vi "SACB - 1.vi"(6 "RH?":bool, 7 "Command":enum16{"Create", "Read", "Close"}(ring), 8 "Error In":errorcluster) -> (0 "Error Out":errorcluster, 3 "Digital Inputs":T1)   [LabVIEW 2017]
uses:
  <vilib>/Modbus/master/Modbus Master.lvclass
  <vilib>/Modbus/master/Create Master Instance (TCP).vi
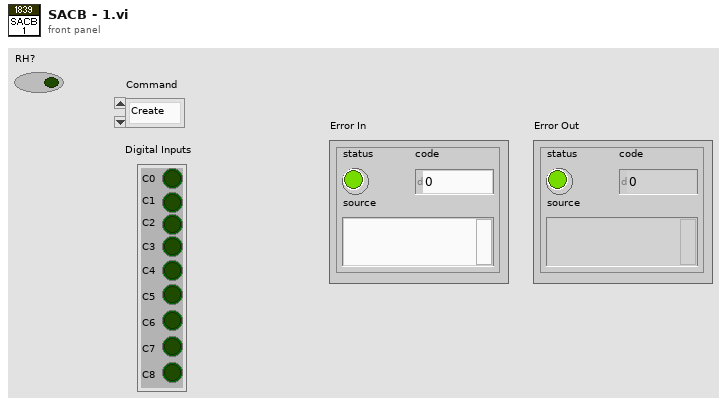
[diagram p1: front panel]
types:
  T1 = cluster{"C0":bool, "C1":bool, "C2":bool, "C3":bool, "C4":bool, "C5":bool, "C6":bool, "C7":bool, "C8":bool}
  T2 = cluster{"Boolean array[0]":bool, "Boolean array[1]":bool, "Boolean array[2]":bool, "Boolean array[3]":bool, "Boolean array[4]":bool, "Boolean array[5]":bool, "Boolean array[6]":bool, "Boolean array[7]":bool, "Boolean array[8]":bool}
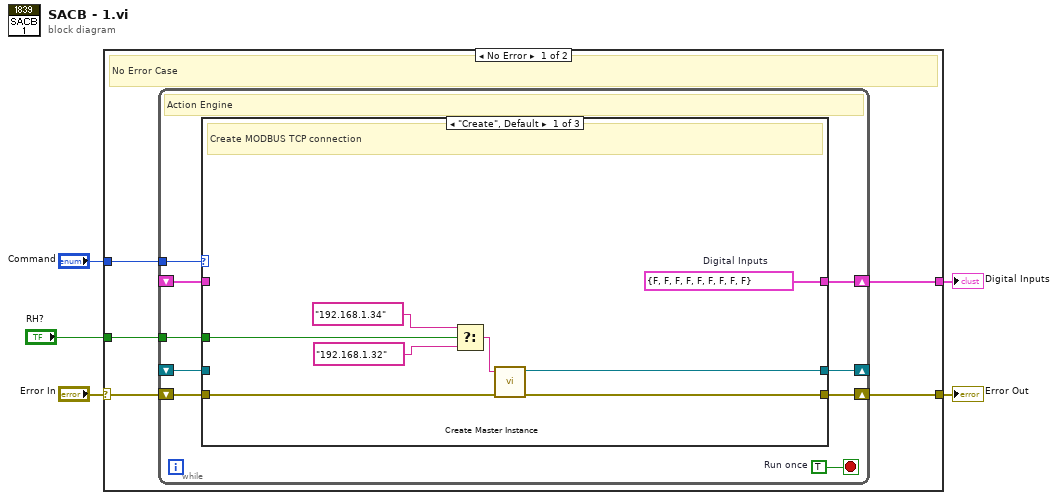
[diagram p0: block diagram]
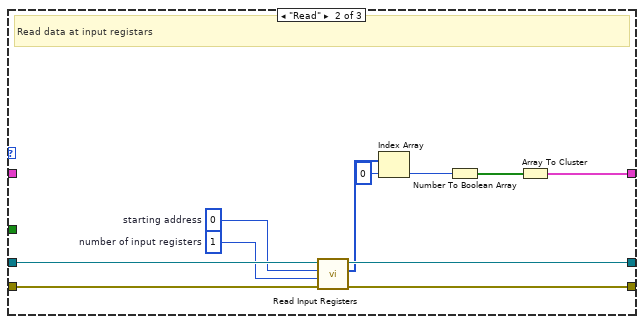
[diagram p2: hidden frame]
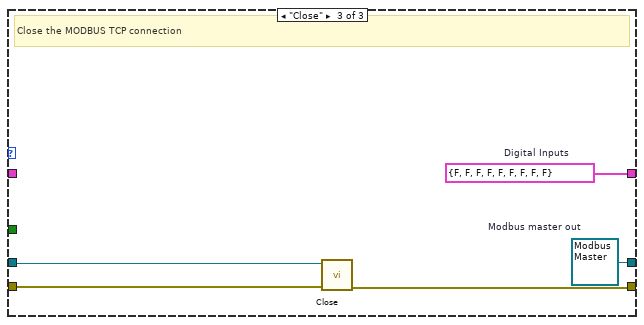
[diagram p3: hidden frame]
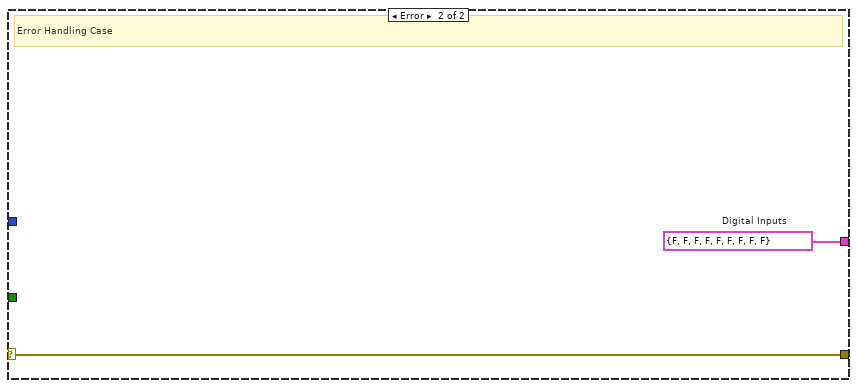
[diagram p4: hidden frame]
diagram:
  n1 = case shown="No Error" "Error In" {
    selector: "Error In" -> [w9 w45]
    tunnel: [w10 w45] -> w4
    tunnel: "Command" -> [w8 _]
    tunnel: [w7 w44] -> w2
    tunnel: "RH?" -> [w6 _]
    frame No Error {
      # "No Error Case"
      n2 = while {
        tunnel: w8 -> [w17]
        shift-right: [w19] -> w10
        shift-left: w9 -> [w18]
        shift-right: [w15] -> _
        shift-left: _ -> [w14]
        shift-right: [w13] -> w7
        shift-left: _ -> [w12]
        tunnel: w6 -> [w11]
        stop <- w16 stop-if-true
        w16 = TRUE  # Run once
        # "Action Engine"
        n3 = case shown="\"Create\", Default" w17 {
          tunnel: [w27 w37 w42] -> w19
          tunnel: w18 -> [w26 w38 w43]
          tunnel: [w25 w36 w40] -> w15
          tunnel: w14 -> [_ w35 w41]
          tunnel: [w24 w28 w39] -> w13
          tunnel: w12 -> [_ _ _]
          tunnel: w11 -> [w22 _ _]
          frame "Create", Default {
            w24 = T1 {"C0"=FALSE, "C1"=FALSE, "C2"=FALSE, "C3"=FALSE, "C4"=FALSE, "C5"=FALSE, "C6"=FALSE, "C7"=FALSE, "C8"=FALSE}  # Digital Inputs
            # "Create MODBUS TCP connection"
            n4 = Select(t="192.168.1.34" ("address"), s=w22, f="192.168.1.32" ("address")) -> (s? t:f=w20:string)
            n5 = call-poly <vilib>:"Create Master Instance.vi"("error in (no error)"=w26, "address"=w20) -> ("error out"=w27:errorcluster, "TCP master instance"=w25:refnum<class "Modbus Master.lvclass">)  [unwired: 8 in]
          }
          frame "Read" {
            w33 = u16 1  # number of input registers
            w34 = u16 0  # starting address
            # "Read data at input registars"
            n6 = call-dynamic "Read Input Registers.vi"("error in (no error)"=w38, "number of input registers"=w33, "starting address"=w34, "Modbus master in"=w35) -> ("error out"=w37:errorcluster, "register values"=w30:u16[], "Modbus master out"=w36:refnum<class "Modbus Master.lvclass">)  [unwired: 5 in]
            n7 = Index Array "Index Array"(array=w30, index=0) -> (element=w31:u16)
            n8 = Number To Boolean Array(number=w31) -> (Boolean array=w32:bool[])
            n9 = Array To Cluster(array=w32) -> (cluster=w28:T2)
          }
          frame "Close" {
            w39 = T1 {"C0"=FALSE, "C1"=FALSE, "C2"=FALSE, "C3"=FALSE, "C4"=FALSE, "C5"=FALSE, "C6"=FALSE, "C7"=FALSE, "C8"=FALSE}  # Digital Inputs
            w40 = refnum<class "Modbus Master.lvclass"> refnum  # Modbus master out
            # "Close the MODBUS TCP connection"
            n10 = call-dynamic "Close.vi"("error in (no error)"=w43, "Modbus master in"=w41) -> ("error out"=w42:errorcluster)  [unwired: 9 in]
          }
        }
      }
    }
    frame Error {
      w44 = T1 {"C0"=FALSE, "C1"=FALSE, "C2"=FALSE, "C3"=FALSE, "C4"=FALSE, "C5"=FALSE, "C6"=FALSE, "C7"=FALSE, "C8"=FALSE}  # Digital Inputs
      # "Error Handling Case"
    }
  }
  "Error Out" <- w4
  "Digital Inputs" <- w2
